vi "Search Array by Name.vi"(0 "Controller Array in":refnum<class "Controller Array.lvclass">, 1 "Name":string) -> (2 "Controller Array Out":refnum<class "Controller Array.lvclass">, 3 "Index of found":i32, 4 "Controller found":refnum<class "Generic Plugin.lvclass">)   [LabVIEW 2020, in "Controller Array.lvclass"]
doc: "Search the array of controllers for one of the same name. This VI will only return the first occurance. If no element was found, it returns an index of -1 and a generic controller object."
uses:
  Controller Array.lvclass
  Controller/Generic Plugin.lvclass
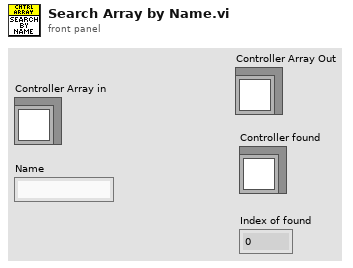
[diagram p1: front panel]
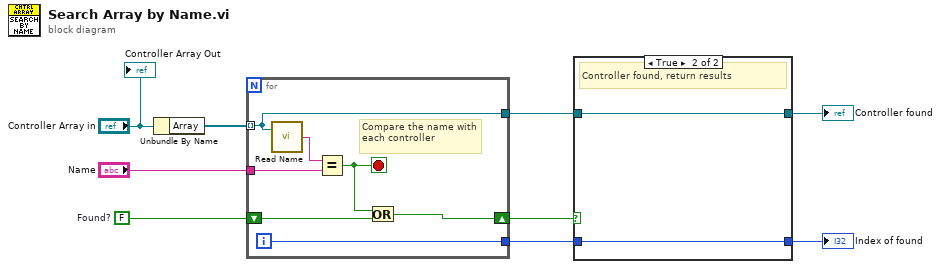
[diagram p0: block diagram]
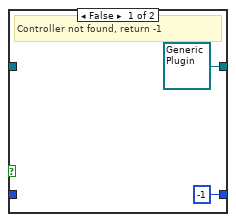
[diagram p2: hidden frame]
diagram:
  w7 = FALSE  # Found?
  n1 = Unbundle By Name("Controller Array in") -> ("Array"=w9:refnum<class "Generic Plugin.lvclass">[])
  n2 = for {
    tunnel: w9 -> [w14] mode=indexing
    tunnel: "Name" -> [w15]
    tunnel: [w14] -> w2
    tunnel: [w13] -> w4
    shift-right: [w11] -> w5
    shift-left: w7 -> [w12]
    i -> [w13]
    stop <- w10 stop-if-true
    # "Compare the name with each controller"
    n3 = call "Read Name.vi"("controller in"=w14) -> ("Name"=w16:string)  [unwired: 1 in, 2 out]
    n4 = Equal?(x=w16, y=w15) -> (x = y?=w10:bool)
    n5 = Or(x=w10, y=w12) -> (x .or. y?=w11:bool)
  }
  n6 = case shown="True" w5 {
    tunnel: [-1 w20] -> w3
    tunnel: w4 -> [_ w20]
    tunnel: w2 -> [_ w19]
    tunnel: [refnum<class "Generic Plugin.lvclass"> refnum ("Controller.lvclass") w19] -> w1
    frame False {
      # "Controller not found, return -1"
    }
    frame True {
      # "Controller found, return results"
    }
  }
  "Index of found" <- w3
  "Controller found" <- w1
  "Controller Array Out" <- "Controller Array in"
